vi "MT_PROTOTYPE.vi"() -> ()   [LabVIEW 2025]
uses:
  CTLs/Producer Cluster.ctl
  CTLs/MAG CLUSTER.ctl
  CTLs/TEMP CLUSTER.ctl
panel:
  in  "stop":bool
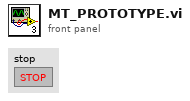
[diagram p1: front panel]
types:
  T1 = typedef "Producer Cluster.ctl" = cluster{"Producer State":enum16{"1. INIT", "2. SET TEMP", "3. WAIT FOR STABILITY (T)", "4. SET FIELD ", "5. WAIT FOR STABILITY (B)", "6. RUN SCAN", "7. RUN BIAS", "8. DRIFT CORRECT (SF)", "9. DRIFT CORRECT (BS)", "10. ADVANCE", "11. SHUTDOWN"}, "Experiment Mode":enum16{"1. SWEEP FIELD", "2. SWEEP TEMP", "3. SWEEP FIELD AND TEMP"}, "Target Temp (K)":dbl[], "Target Field (T)":dbl[], "Temp Index":i32, "Field Index":i32, "Current Temp":dbl, "Current Field":dbl}
  T2 = enum16{"1. INIT", "2. SET TEMP", "3. WAIT FOR STABILITY (T)", "4. SET FIELD ", "5. WAIT FOR STABILITY (B)", "6. RUN SCAN", "7. RUN BIAS", "8. DRIFT CORRECT (SF)", "9. DRIFT CORRECT (BS)", "10. ADVANCE", "11. SHUTDOWN"}
  T3 = enum16{"1. TEMP STABLE", "2. FIELD STABLE", "3. SCAN DONE", "4. BIAS DONE", "5. DRIFT CORRECTED (SF)", "6. DRIFT CORRECTED (BS)"}
  T4 = enum16{"1. INIT MAG", "2. PREP FIELD", "3. APPLY FIELD", "4. MAG STAB", "5. MAG IDLE", "6. MAG OFF"}
  T5 = typedef "MAG CLUSTER.ctl" = cluster{"Ramp Target":enum16{"ZERO", "MID", "MAX"}, "Pause":bool, "Switch Heater":bool, "Persistent Field":dbl, "Persistent Current":dbl, "Tesla":bool, "Output (T)":dbl, "Output (A)":dbl, "X Trip":enum16{"DISABLED", "ENABLED", "ACTIVE"}, "Ramp Rate (A/s)":dbl, "V Limit (V)":dbl, "Heater Voltage":dbl, "MAX Setpoint (A)":dbl, "MAX Setpoint (T)":dbl, "MID Setpoint (A)":dbl, "MID Setpoint (T)":dbl, "Lock":bool, "Field Constant":dbl, "Remote":bool, "Direction":enum16{"POSITIVE", "NEGATIVE", "OPEN", "UNIPOLAR"}, "Helium Level":u16, "Quench !":bool, "Voltage":dbl, "V Limit !":bool, "Ramping":bool, "At Target":bool, "Trip Field":dbl, "Trip Current":dbl, "Current State":enum16{"1. INIT MAG", "2. PREP FIELD", "3. APPLY FIELD", "4. MAG STAB", "5. MAG IDLE", "6. MAG OFF"}, "MAG Reference":refnum<visa-resource-name>}
  T6 = enum16{"1. INIT_TEMP", "2. SET_TEMP", "3. WAIT_STABLE", "4. TEMP_IDLE", "5. TC OFF (Reset)"}
  T7 = typedef "TEMP CLUSTER.ctl" = cluster{"Range (0:Off)":u16, "Manual Output (0.00 %)":dbl, "Rate (D) (0.0 %)":dbl, "Reset (I) (20.0)":dbl, "Gain (P) (50.0)":dbl, "Power Up Enable (F: Disable)":bool, "Max User Current (2.000)":dbl, "Heater Resistance (1:25 Ohms)":u16, "Max Current (0:User Specified)":u16, "Heater Out Display (1:Current)":u16, "Mode (0:Off)":u16, "Input (0:None)":u16, "Target Temp (K)":dbl, "Serial Configuration":cluster{"Baud Rate":u32, "Parity":u16, "Data Bits":u16, "Stop Bits":u16, "Flow Control":u16}, "VISA resource name":refnum<visa-resource-name>, "Configure Control Parameters (0: Configure)":u16, "Enable Setpoint (F:Disable)":bool, "Input (0:A)":u16, "Data Source (0:Kelvin)":u16, "Output's Control Loop (1:1)":u16, "STND DEV Threshold ":dbl, "Mean Tolerance ":dbl, "Current State":enum16{"1. INIT_TEMP", "2. SET_TEMP", "3. WAIT_STABLE", "4. TEMP_IDLE", "5. TC OFF (Reset)"}}
  T8 = typedef "ACK Cluster.ctl" = cluster{"ACK States":enum16{"1. TEMP STABLE", "2. FIELD STABLE", "3. SCAN DONE", "4. BIAS DONE", "5. DRIFT CORRECTED (SF)", "6. DRIFT CORRECTED (BS)"}, "Drift Correction Values":dbl[][]}
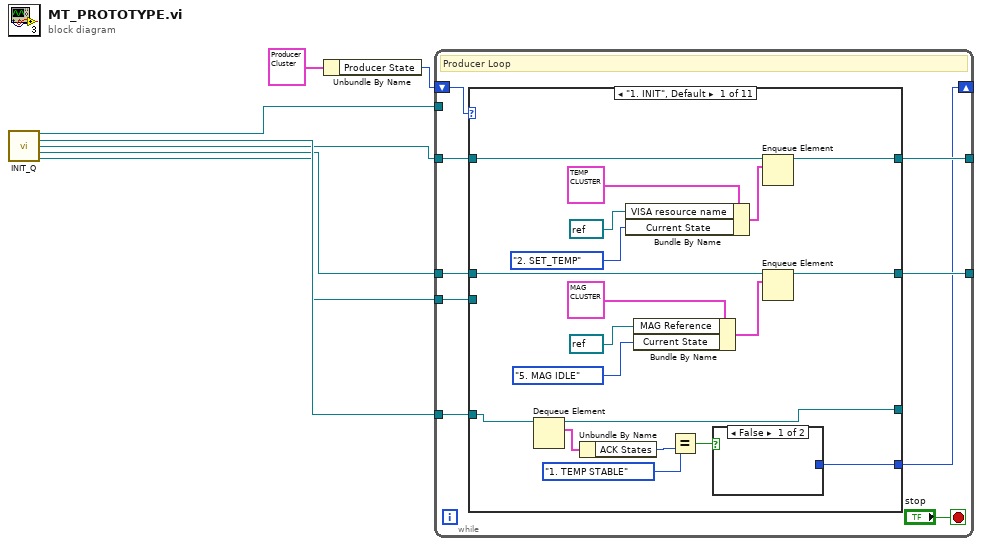
[diagram p0: block diagram]
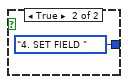
[diagram p2: hidden frame]
diagram:
  n1 = call "INIT_Q.vi"() -> ("MainQ Out"=w3:refnum<queue>, "ACKQ Out"=w7:refnum<queue>, "TempQ Out"=w6:refnum<queue>, "MagQ Out"=w5:refnum<queue>, "ScanQ Out"=w4:refnum<queue>)  [unwired: 11 in]
  n2 = Unbundle By Name(T1 {"Producer State"=enum."1. INIT", "Experiment Mode"=enum."1. SWEEP FIELD", "Target Temp (K)"=[], "Target Field (T)"=[], "Temp Index"=0, "Field Index"=0, "Current Temp"=0.0, "Current Field"=0.0} ("Producer Cluster")) -> ("Producer State"=w1:T2)
  n3 = while {
    tunnel: w7 -> [w15]
    tunnel: w6 -> [w14]
    tunnel: w5 -> [w13]
    tunnel: w4 -> [w12]
    tunnel: w3 -> [_]
    shift-right: [w9] -> _
    shift-left: w1 -> [w16]
    tunnel: [w11] -> _
    tunnel: [w10] -> _
    stop <- "stop" stop-if-true
    # "Producer Loop"
    n4 = case shown="\"1. INIT\", Default" w16 {
      tunnel: w15 -> [w23 _ _ _ _ _ _ _ _ _ _]
      tunnel: w14 -> [w35 _ _ _ _ _ _ _ _ _ _]
      tunnel: w13 -> [w34 _ _ _ _ _ _ _ _ _ _]
      tunnel: w12 -> [_ _ _ _ _ _ _ _ _ _ _]
      tunnel: [w29 _ _ _ _ _ _ _ _ _ _] -> w11
      tunnel: [w24 _ _ _ _ _ _ _ _ _ _] -> w10
      tunnel: [w20 _ _ _ _ _ _ _ _ _ _] -> _
      tunnel: [w17 _ _ _ _ _ _ _ _ _ _] -> w9
      frame "1. INIT", Default {
        n5 = Dequeue Element(queue=w23) -> (queue out=w20:refnum<queue>, element=w22:T8)  [unwired: 2 in, 2 out]
        n6 = Unbundle By Name(w22) -> ("ACK States"=w21:T3)
        n7 = Bundle By Name(cluster=T7 {"Range (0:Off)"=0, "Manual Output (0.00 %)"=0.0, "Rate (D) (0.0 %)"=0.0, "Reset (I) (20.0)"=20.0, "Gain (P) (50.0)"=50.0, "Power Up Enable (F: Disable)"=FALSE, "Max User Current (2.000)"=2.0, "Heater Resistance (1:25 Ohms)"=1, "Max Current (0:User Specified)"=0, "Heater Out Display (1:Current)"=1, "Mode (0:Off)"=1, "Input (0:None)"=4, "Target Temp (K)"=5.0, "Serial Configuration"={"Baud Rate"=57600, "Parity"=1, "Data Bits"=7, "Stop Bits"=10, "Flow Control"=0}, "VISA resource name"="", "Configure Control Parameters (0: Configure)"=0, "Enable Setpoint (F:Disable)"=FALSE, "Input (0:A)"=3, "Data Source (0:Kelvin)"=0, "Output's Control Loop (1:1)"=2, "STND DEV Threshold "=0.1, "Mean Tolerance "=0.01, "Current State"=enum."1. INIT_TEMP"} ("Temp Controller"), "VISA resource name"=refnum<visa-resource-name> refnum, "Current State"=T6."2. SET_TEMP") -> (w30:T7)
        n8 = Bundle By Name(cluster=T5 {"Ramp Target"=enum."ZERO", "Pause"=FALSE, "Switch Heater"=FALSE, "Persistent Field"=0.0, "Persistent Current"=0.0, "Tesla"=FALSE, "Output (T)"=0.0, "Output (A)"=0.0, "X Trip"=enum."DISABLED", "Ramp Rate (A/s)"=0.0, "V Limit (V)"=0.0, "Heater Voltage"=0.0, "MAX Setpoint (A)"=0.0, "MAX Setpoint (T)"=0.0, "MID Setpoint (A)"=0.0, "MID Setpoint (T)"=0.0, "Lock"=FALSE, "Field Constant"=0.0, "Remote"=FALSE, "Direction"=enum."POSITIVE", "Helium Level"=0, "Quench !"=FALSE, "Voltage"=0.0, "V Limit !"=FALSE, "Ramping"=FALSE, "At Target"=FALSE, "Trip Field"=0.0, "Trip Current"=0.0, "Current State"=enum."1. INIT MAG", "MAG Reference"="COM4"} ("PSU Status In"), "MAG Reference"=refnum<visa-resource-name> refnum, "Current State"=T4."5. MAG IDLE") -> (w27:T5)
        n9 = Equal?(x=T3."1. TEMP STABLE", y=w21) -> (x = y?=w18:bool)
        n10 = case shown="False" w18 {
          tunnel: [_ T2."4. SET FIELD " ("Producer State")] -> w17
          frame False {
          }
          frame True {
          }
        }
        n11 = Enqueue Element(queue=w35, element=w30) -> (queue out=w29:refnum<queue>)  [unwired: 2 in, 2 out]
        n12 = Enqueue Element(queue=w34, element=w27) -> (queue out=w24:refnum<queue>)  [unwired: 2 in, 2 out]
      }
      frame "2. SET TEMP" {
      }
      frame "3. WAIT FOR STABILITY (T)" {
      }
      frame "4. SET FIELD " {
      }
      frame "5. WAIT FOR STABILITY (B)" {
      }
      frame "6. RUN SCAN" {
      }
      frame "7. RUN BIAS" {
      }
      frame "8. DRIFT CORRECT (SF)" {
      }
      frame "9. DRIFT CORRECT (BS)" {
      }
      frame "10. ADVANCE" {
      }
      frame "11. SHUTDOWN" {
      }
    }
  }
